vi "Initialize Driver.vi"(8 "error in (no error)":errorcluster, 10 "Section Ref in":T21 format="%.0x", 11 "Plugin in":refnum<class "Plugin.lvclass">) -> (0 "error out":errorcluster, 2 "Vars":T1 {"OutgoingRegisters.Refs"."Data Type" format="%.0x"; "IncomingDMA.Refs"."Refs"."Data Type" format="%.0x"; "IncomingDMA.Refs"."DMA Settings"."DMA Host Buffer" items=["1 Second"=1, "2 Seconds"=2, "5 Seconds"=5, "10 Seconds"=10]; "IncomingDMA.Refs"."DMA Settings"."dt" format="%#_p"; "IncomingDMA.Refs"."DMA Settings"."Update Rate" items=["1 Hz"=1, "2 Hz"=2, "5 Hz"=5, "10 Hz"=10]; "IncomingRegisters.Refs"."Data Type" format="%.0x"; "OutgoingDMA.Refs"."Refs"."Data Type" format="%.0x"; "Compiled"."IncomingRegisters.Settings"."Register"."Data Type" format="%.0x"; "Compiled"."IncomingRegisters.Refs"."Refs"."Data Reference" format="%.0x"; "Compiled"."OutgoingRegisters.Settings"."Register"."Data Type" format="%.0x"; "Compiled"."OutgoingRegisters.Refs"."Refs"."Data Reference" format="%.0x"; "Compiled"."IncomingDMA.Settings"."Data Type" format="%.0x"; "Compiled"."IncomingDMA.Settings"."DMA.Settings"."DMA Host Buffer" items=["1 Second"=1, "2 Seconds"=2, "5 Seconds"=5, "10 Seconds"=10]; "Compiled"."IncomingDMA.Settings"."DMA.Settings"."dt" format="%#_p"; "Compiled"."IncomingDMA.Settings"."DMA.Settings"."Update Rate" items=["1 Hz"=1, "2 Hz"=2, "5 Hz"=5, "10 Hz"=10]; "Compiled"."OutgoingDMA.Settings"."Data Type" format="%.0x"; "Compiled"."OutgoingDMA.Settings"."DMA.Settings"."DMA Host Buffer" items=["1 Second"=1, "2 Seconds"=2, "5 Seconds"=5, "10 Seconds"=10]; "Compiled"."OutgoingDMA.Settings"."DMA.Settings"."dt" format="%#_p"; "Compiled"."OutgoingDMA.Settings"."DMA.Settings"."Update Rate" items=["1 Hz"=1, "2 Hz"=2, "5 Hz"=5, "10 Hz"=10]}, 3 "Plugin out":refnum<class "Plugin.lvclass">)   [LabVIEW 2024, in "FPGA Addon Engine.lvlib" / "Plugin.lvclass"]
uses:
  Plugin.lvclass
  Plugin.lvclass/Plugin.ctl
  Addon Shared/Types/FG Action.ctl
  Addon Shared/FPGA Addon Shared.lvlib
  <vilib>/NI VeriStand/Custom Device API/Custom Device Target Type.ctl
  <vilib>/NI VeriStand/Custom Device API/Custom Device API.lvlib
  Addon Shared/Types/FPGA Settings.ctl
  <vilib>/NI VeriStand/Custom Device API/Waveform Data Reference.ctl
  Addon Shared/Types/DMA Acquisition Mode.ctl
  Addon Shared/Types/Delacing Scheme.ctl
  Addon Shared/Types/DMA Settings.ctl
  Addon Shared/Types/FPGA Addon Data Type.ctl
  Addon Shared/Types/Compiled.DMASettings.ctl
  <vilib>/NI VeriStand/Custom Device API/Data Reference.ctl
  <vilib>/NI VeriStand/Custom Device API/Block Data Reference.ctl
  Addon Shared/Types/Register Information.ctl
  Addon Shared/Types/Scalar Type.ctl
  Addon Shared/Types/Compiled.RegisterSettings.ctl
  Addon Shared/Types/Compiled.Settings.ctl
  Types/DMA Output Refs.ctl
  FPGA Addon Engine.lvlib
  <vilib>/NI VeriStand/Custom Device Waveform API/Single Waveform Read (DBL)/Single Waveform Read (DBL).lvclass
  Types/DMA Output References.ctl
  Types/Register Settings.ctl
  Types/DMA Input Refs.ctl
  <vilib>/NI VeriStand/Custom Device Waveform API/Multiple Waveforms Write (DBL)/Multiple Waveforms Write (DBL).lvclass
  Types/DMA Input References.ctl
  Types/State Variables.ctl
  APIs/FPGA Register IO/FPGA Register IO.lvlib
  Addon Shared/SubVIs/Constants.vi
  <vilib>/NI VeriStand/Custom Device API/Get Item Property (Variant).vi
  <vilib>/NI VeriStand/Custom Device API/Get Item Property (Dependent File).vi
  <vilib>/NI VeriStand/Custom Device API/Custom Device Item Ref.ctl
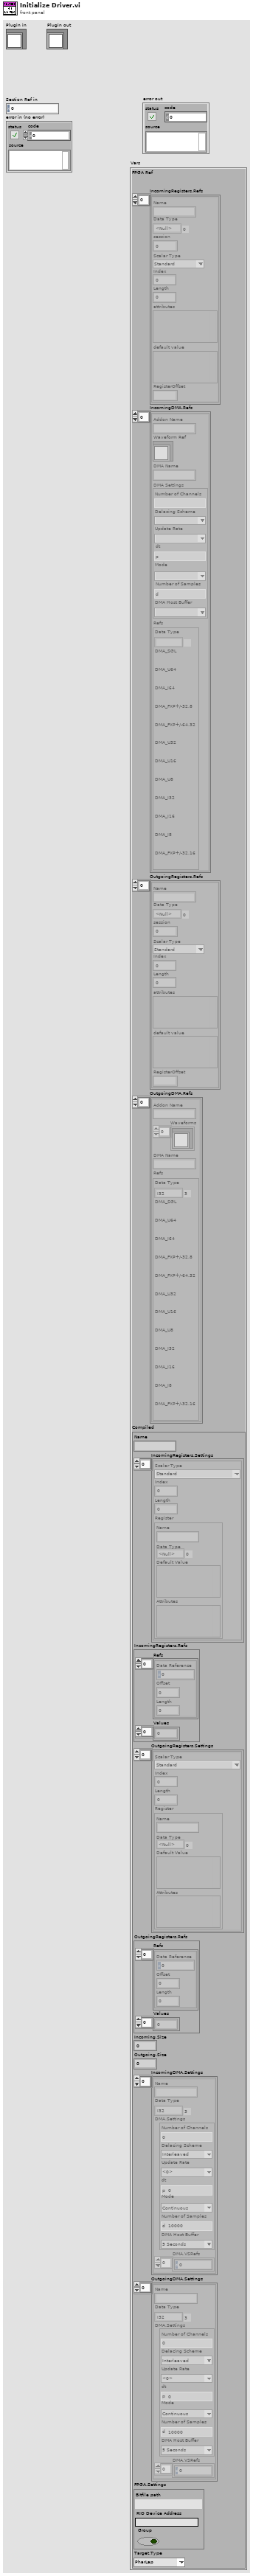
[diagram p1: front panel]
types:
  T1 = typedef "FPGA Addon Engine.lvlib/State Variables.ctl" = cluster{"FPGA Ref":refnum<k20>, "IncomingRegisters.Refs":T2[], "IncomingDMA.Refs":T5[], "OutgoingRegisters.Refs":T2[], "OutgoingDMA.Refs":T10[], "Compiled":T12}
  T2 = typedef "FPGA Addon Engine.lvlib/Register Settings.ctl" = cluster{"Name":string, "Data Type":T3, "session":u32, "Scalar Type":T4, "Index":i32, "Length":i32, "attributes":variant, "default value":variant, "RegisterOffset":u32}
  T3 = typedef "FPGA Addon Shared.lvlib/FPGA Addon Data Type.ctl" = enum8{"<Null>", "I8", "I16", "I32", "I64", "U8", "U16", "U32", "U64", "SGL", "Boolean", "Analog PWM In Settings", "Analog PWM In", "Digital PWM In Settings", "Digital PWM In", "Digital PWM Out", "Sine Out", "FXP", "FXP+/-24.5", "FXP+/-16.5", "FXP+/-32.8", "FXP+/-64.32", "FXP+/-16.7", "FXP+/-20.5", "FXP+/-27.5", "FXP+/-32.16", "FXP+16.3", "FXP+18.3", "Digital Static In", "Digital Static Out", "Digital Static In Settings", "Digital WSS Out", "Quad Encoder Settings", "Quad Encoder In", "Group"}
  T4 = typedef "FPGA Addon Shared.lvlib/Scalar Type.ctl" = enum16{"Standard", "Bitpacked"}
  T5 = typedef "FPGA Addon Engine.lvlib/DMA Input References.ctl" = cluster{"Addon Name":string, "Waveform Ref":refnum<class "Multiple Waveforms Write (DBL).lvclass">, "DMA Name":string, "DMA Settings":T6, "Refs":T9}
  T6 = typedef "FPGA Addon Shared.lvlib/DMA Settings.ctl" = cluster{"Number of Channels":u8, "Delacing Scheme":T7, "Update Rate":u32, "dt":dbl, "Mode":T8, "Number of Samples":u32, "DMA Host Buffer":u32}
  T7 = typedef "FPGA Addon Shared.lvlib/Delacing Scheme.ctl" = enum8{"Interleaved", "Bitpacked"}
  T8 = typedef "FPGA Addon Shared.lvlib/DMA Acquisition Mode.ctl" = enum8{"Continuous", "Triggered Finite"}
  T9 = typedef "FPGA Addon Engine.lvlib/DMA Input Refs.ctl" = cluster{"Data Type":T3, "DMA_SGL":refnum<k20>, "DMA_U64":refnum<k20>, "DMA_I64":refnum<k20>, "DMA_FXP+/-32.8":refnum<k20>, "DMA_FXP+/-64.32":refnum<k20>, "DMA_U32":refnum<k20>, "DMA_U16":refnum<k20>, "DMA_U8":refnum<k20>, "DMA_I32":refnum<k20>, "DMA_I16":refnum<k20>, "DMA_I8":refnum<k20>, "DMA_FXP+/-32.16":refnum<k20>}
  T10 = typedef "FPGA Addon Engine.lvlib/DMA Output References.ctl" = cluster{"Addon Name":string, "Waveforms":refnum<class "Single Waveform Read (DBL).lvclass">[], "DMA Name":string, "Refs":T11}
  T11 = typedef "FPGA Addon Engine.lvlib/DMA Output Refs.ctl" = cluster{"Data Type":T3, "DMA_SGL":refnum<k20>, "DMA_U64":refnum<k20>, "DMA_I64":refnum<k20>, "DMA_FXP+/-32.8":refnum<k20>, "DMA_FXP+/-64.32":refnum<k20>, "DMA_U32":refnum<k20>, "DMA_U16":refnum<k20>, "DMA_U8":refnum<k20>, "DMA_I32":refnum<k20>, "DMA_I16":refnum<k20>, "DMA_I8":refnum<k20>, "DMA_FXP+/-32.16":refnum<k20>}
  T12 = typedef "FPGA Addon Shared.lvlib/Compiled.Settings.ctl" = cluster{"Name":string, "IncomingRegisters.Settings":T13[], "IncomingRegisters.Refs":cluster{"Refs":T15[], "Values":dbl[]}, "OutgoingRegisters.Settings":T13[], "OutgoingRegisters.Refs":cluster{"Refs":T15[], "Values":dbl[]}, "Incoming.Size":i32, "Outgoing.Size":i32, "IncomingDMA.Settings":T17[], "OutgoingDMA.Settings":T17[], "FPGA.Settings":T19, "Target.Type":T20}
  T13 = typedef "FPGA Addon Shared.lvlib/Compiled.RegisterSettings.ctl" = cluster{"Scalar Type":T4, "Index":i32, "Length":i32, "Register":T14}
  T14 = typedef "FPGA Addon Shared.lvlib/Register Information.ctl" = cluster{"Name":string, "Data Type":T3, "Default Value":variant, "Attributes":variant}
  T15 = typedef "Custom Device API.lvlib/Block Data Reference.ctl" = cluster{"Data Reference":T16, "Offset":u64, "Length":u64}
  T16 = typedef "Custom Device API.lvlib/Data Reference.ctl" = i32
  T17 = typedef "FPGA Addon Shared.lvlib/Compiled.DMASettings.ctl" = cluster{"Name":string, "Data Type":T3, "DMA.Settings":T6, "DMA.VSRefs":T18[]}
  T18 = typedef "Custom Device API.lvlib/Waveform Data Reference.ctl" = i32
  T19 = typedef "FPGA Addon Shared.lvlib/FPGA Settings.ctl" = cluster{"Bitfile path":path, "RIO Device Address":string, "Group":bool}
  T20 = typedef "Custom Device API.lvlib/Custom Device Target Type.ctl" = enum16{"PharLap", "VxWorks", "Windows", "Linux_32_ARM", "Linux_x64"}
  T21 = typedef "Custom Device API.lvlib/Custom Device Item Ref.ctl" = u64
  T22 = typedef "FPGA Addon Shared.lvlib/FG Action.ctl" = enum8{"GET", "SET"}
  T23 = typedef "Custom Device API.lvlib/Dependent File Optional Info.ctl" = cluster{"Version":string, "RTDestination":path, "ForceDownload":bool, "SupportedTarget":string, "MD5":string}
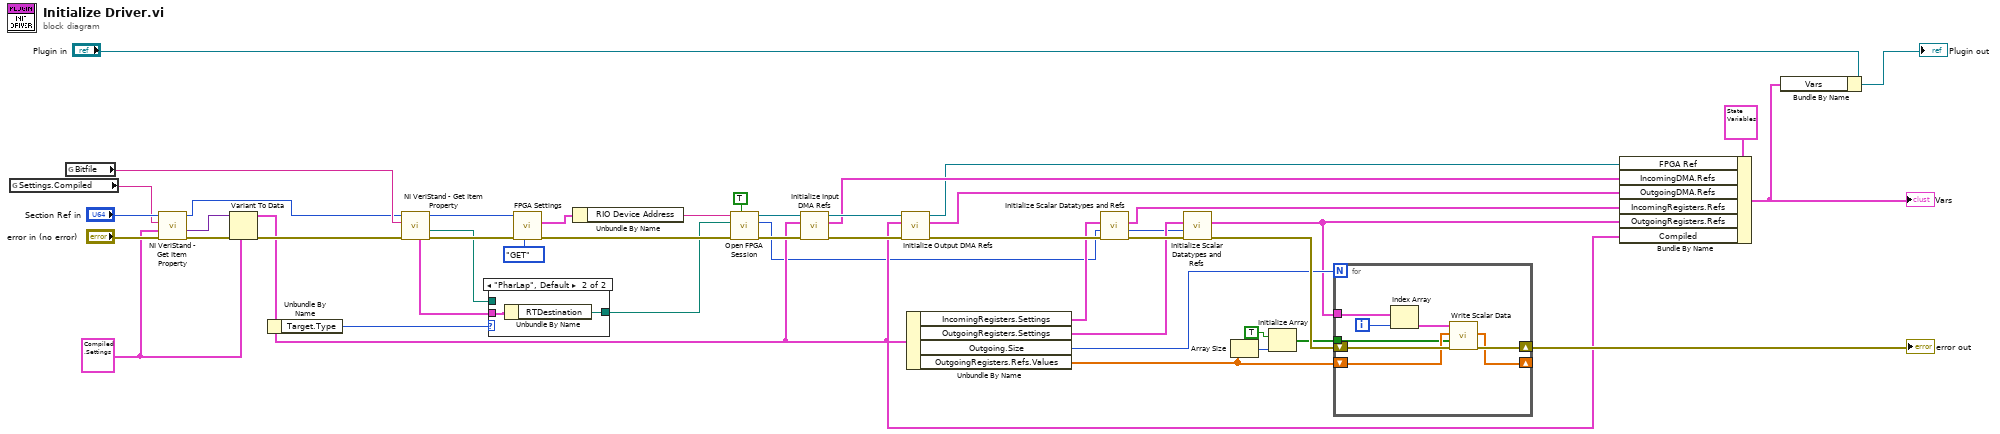
[diagram p0: block diagram]
diagram:
  w20 = T12 {"Name"="", "IncomingRegisters.Settings"=[], "IncomingRegisters.Refs"={"Refs"=[], "Values"=[]}, "OutgoingRegisters.Settings"=[], "OutgoingRegisters.Refs"={"Refs"=[], "Values"=[]}, "Incoming.Size"=0, "Outgoing.Size"=0, "IncomingDMA.Settings"=[], "OutgoingDMA.Settings"=[], "FPGA.Settings"={"Bitfile path"=path "", "RIO Device Address"="", "Group"=FALSE}, "Target.Type"=enum."PharLap"} ("Settings.Compiled")
  n1 = global read "Constants.vi" "Settings.Compiled"() -> (w22:string)
  n2 = global read "Constants.vi" "Bitfile"() -> (w33:string)
  n3 = call-poly <vilib>:"NI VeriStand - Get Item Property.vi"("error in (no error)"="error in (no error)", "Default Value"=w20, "Property Name"=w22, "Item Ref in"="Section Ref in") -> ("error out"=w43:errorcluster, "Value"=w21:variant, "Item Ref out"=w17:T21)  [unwired: 4 in, 1 out]
  n4 = Variant To Data(error in=w43, type=w20, Variant=w21) -> (data=w19:T12, error out=w42:errorcluster)
  n5 = Unbundle By Name(w19) -> ("Target.Type"=w18:T20)
  n6 = call-poly <vilib>:"NI VeriStand - Get Item Property.vi"("error in (no error)"=w42, "Property Name"=w33, "Item Ref in"=w17) -> ("error out"=w47:errorcluster, "Path"=w30:path, "Item Ref out"=w32:T21, "OptionalInfo"=w31:T23)  [unwired: 4 in, 1 out]
  n7 = case shown="\"PharLap\", Default" w18 {
    tunnel: w31 -> [_ w50]
    tunnel: [w48 w49] -> w10
    tunnel: w30 -> [w48 _]
    frame "Windows" {
    }
    frame "PharLap", Default {
      n8 = Unbundle By Name(w50) -> ("RTDestination"=w49:path)
    }
  }
  n9 = call "FPGA Settings.vi"("Action"=FG_Action."GET", "error in (no error)"=w47, "Item Ref"=w32) -> ("error out"=w38:errorcluster, "FPGA Settings"=w35:T19)  [unwired: 6 in, 1 out]
  n10 = Unbundle By Name(w35) -> ("RIO Device Address"=w11:string)
  n11 = call "Open FPGA Session.vi"("run when loaded (T)"=TRUE ("Run When Loaded"), "error in"=w38, "bitfile path"=w10, "device address"=w11) -> ("error out"=w37:errorcluster, "session out"=w6:u32, "bitfile reference out"=w9:refnum<k20>)  [unwired: 5 in]
  n12 = call "Initialize Input DMA Refs.vi"("error in (no error)"=w37, "Settings.Compiled"=w19, "FPGA Ref"=w9) -> ("error out"=w45:errorcluster, "DMA Settings"=w26:T5[], "FPGA Ref"=w27:refnum<k20>)  [unwired: 6 in]
  n13 = call "Initialize Output DMA Refs.vi"("error in (no error)"=w45, "Settings.Compiled"=w19, "FPGA Ref"=w27) -> ("error out"=w46:errorcluster, "DMA"=w25:T10[], "FPGA Ref"=w5:refnum<k20>)  [unwired: 6 in]
  n14 = Unbundle By Name(w19) -> ("IncomingRegisters.Settings"=w29:T13[], "OutgoingRegisters.Settings"=w28:T13[], "Outgoing.Size"=w14:i32, "OutgoingRegisters.Refs.Values"=w13:dbl[])
  n15 = call "Initialize Scalar Datatypes and Refs.vi"("error in (no error)"=w46, "session in"=w6, "Registers"=w29) -> ("error out"=w40:errorcluster, "session out"=w4:u32, "Registers Ref"=w24:T2[])  [unwired: 6 in]
  n16 = call "Initialize Scalar Datatypes and Refs.vi"("error in (no error)"=w40, "session in"=w4, "Registers"=w28) -> ("error out"=w39:errorcluster, "Registers Ref"=w7:T2[])  [unwired: 6 in, 1 out]
  n17 = Array Size(array=w13) -> (size(s)=w12:i32)
  n18 = Initialize Array(TRUE, w12) -> (w15:bool[])
  n19 = for {
    N: w14 -> [_]
    shift-right: [w54] -> _
    shift-left: w13 -> [w55]
    shift-right: [w57] -> w41
    shift-left: w39 -> [w58]
    tunnel: w15 -> [w53]
    tunnel: w7 -> [w51]
    i -> [w52]
    n20 = Index Array(array=w51, index=w52) -> (element=w56:T2)
    n21 = call "Write Scalar Data.vi"("error in (no error)"=w58, "Changed?"=w53, "Values"=w55, "Cluster"=w56) -> ("error out"=w57:errorcluster, "Values"=w54:dbl[])  [unwired: 6 in]
  }
  "error out" <- w41
  n22 = Bundle By Name(cluster=T1 {"FPGA Ref"=refnum, "IncomingRegisters.Refs"=[], "IncomingDMA.Refs"=[], "OutgoingRegisters.Refs"=[], "OutgoingDMA.Refs"=[], "Compiled"={"Name"="", "IncomingRegisters.Settings"=[], "IncomingRegisters.Refs"={"Refs"=[], "Values"=[]}, "OutgoingRegisters.Settings"=[], "OutgoingRegisters.Refs"={"Refs"=[], "Values"=[]}, "Incoming.Size"=0, "Outgoing.Size"=0, "IncomingDMA.Settings"=[], "OutgoingDMA.Settings"=[], "FPGA.Settings"={"Bitfile path"=path "", "RIO Device Address"="", "Group"=FALSE}, "Target.Type"=enum."PharLap"}}, "FPGA Ref"=w5, "IncomingDMA.Refs"=w26, "OutgoingDMA.Refs"=w25, "IncomingRegisters.Refs"=w24, "OutgoingRegisters.Refs"=w7, "Compiled"=w19) -> (w3:T1)
  "Vars" <- w3
  n23 = Bundle By Name(cluster="Plugin in", "Vars"=w3) -> (→"Plugin out":refnum<class "Plugin.lvclass">)
